vi "main.vi"() -> ()   [LabVIEW 2011, in "ttmServer.lvclass"]
uses:
  ttmServer.lvclass
  ttmServer.lvclass/ttmServer.ctl
panel:
  in  "Front panel name":u16(ring)=3 items=["viewer", "ttm_aecontrol_poller.vi", "ttm_creep_poller.vi", "ttm_lightIndicator_poller.vi", "ttm_logging_poller.vi", "ttm_moveToSetpoint_poller.vi", "ttm_status_poller.vi", "ttm_stop_poller.vi", "ttm_tensile_poller.vi", "ttm_tensilecyclic_poller.vi", "ttm_variableCalculator_poller.vi", "ttm_variableSaver_poller.vi"]
  in  "stop":bool
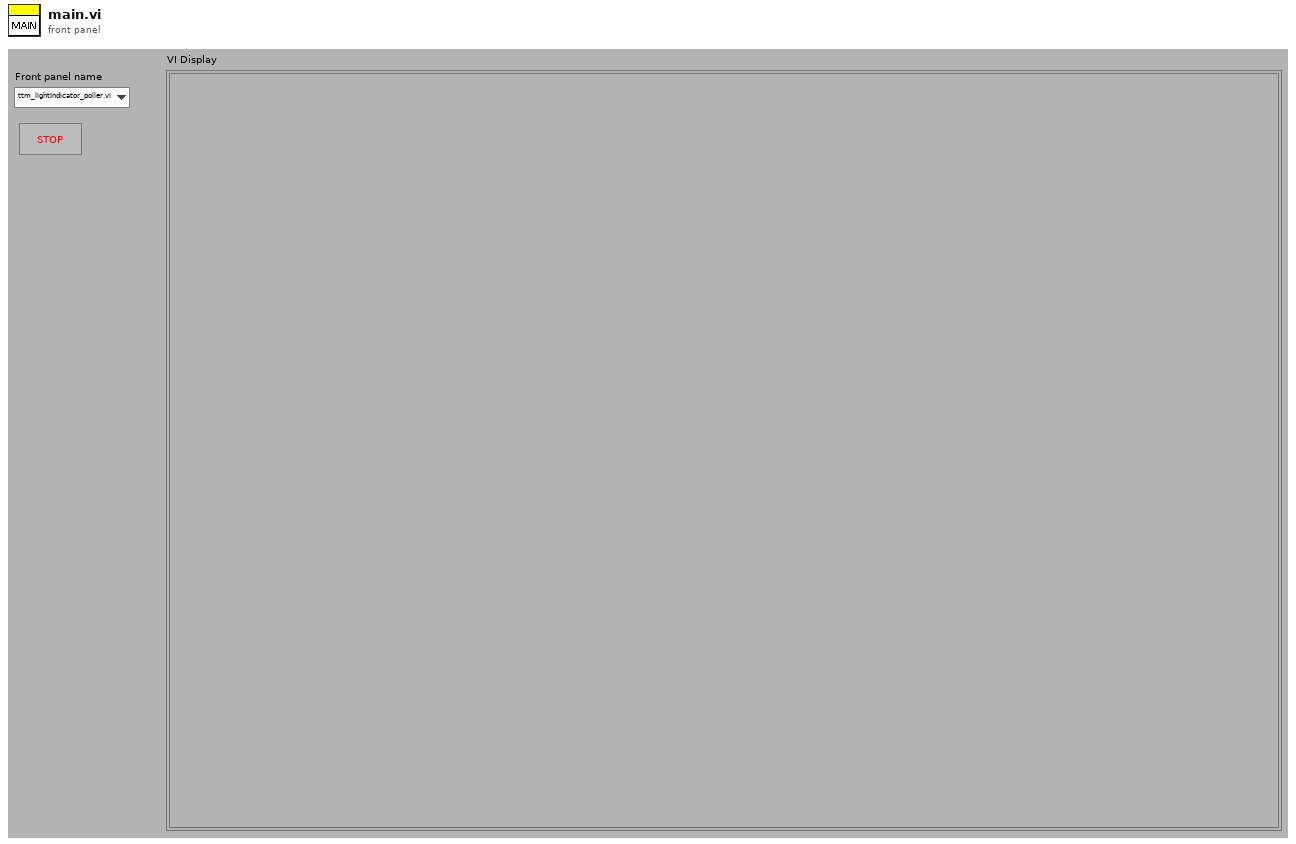
[diagram p1: front panel]
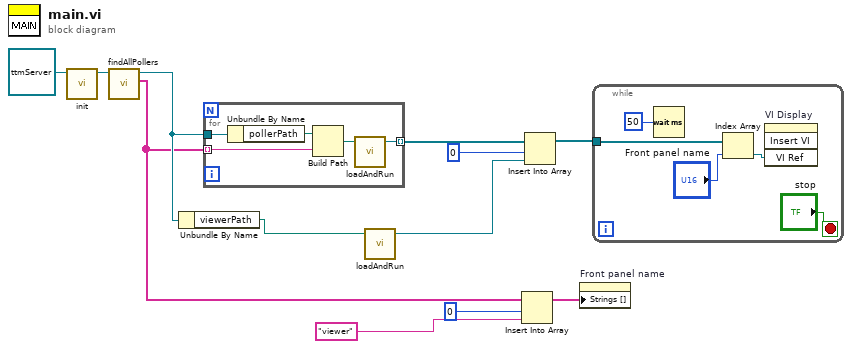
[diagram p0: block diagram]
diagram:
  n1 = call "init.vi"("ttm_poller_panel.vi.lvclass"=refnum<class "ttmServer.lvclass"> refnum ("ttm_poller_panel.vi.lvclass 3")) -> ("output cluster"=w11:refnum<class "ttmServer.lvclass">)  [unwired: 10 in]
  n2 = call "findAllPollers.vi"("ttm_poller_panel_in"=w11) -> ("pollerFileNames"=w3:string[], "ttm_poller_panel_out"=w7:refnum<class "ttmServer.lvclass">)  [unwired: 9 in]
  n3 = Unbundle By Name(w7) -> ("viewerPath"=w6:path)
  n4 = for {
    tunnel: [w17] -> w10 mode=indexing
    tunnel: w7 -> [w16]
    tunnel: w3 -> [w14] mode=indexing
    n5 = Unbundle By Name(w16) -> ("pollerPath"=w15:path)
    n6 = Build Path(base path=w15, name or relative path=w14) -> (appended path=w13:path)
    n7 = call "loadAndRun.vi"("path"=w13) -> ("vi refnum out"=w17:refnum<vi>)  [unwired: 3 in, 1 out]
  }
  n8 = call "loadAndRun.vi"("path"=w6) -> ("vi refnum out"=w8:refnum<vi>)  [unwired: 3 in, 1 out]
  n9 = Insert Into Array(array=w3, index=0, new element="viewer" ("new element/subarray")) -> (w1:string[])
  n10 = Insert Into Array(array=w10, index=0, new element=w8) -> (w5:refnum<vi>[])
  n11 = property on="Front panel name" class="Ring (strict)"("Strings []"=w1) -> ()  [unwired: 2 in, 2 out]
  n12 = while {
    tunnel: w5 -> [w20]
    stop <- "stop" stop-if-true
    n13 = Wait (ms)(milliseconds to wait=50) -> ()  [unwired: 1 out]
    n14 = Index Array(array=w20, index="Front panel name") -> (element=w19:refnum<vi>)
    n15 = invoke on="VI Display" class="SubPnl" method="Insert VI"("VI Ref"=w19) -> ()  [unwired: 3 in, 4 out]
  }
